vi "GetPathFromTimeStamp.vi"(2 "UTC Time":bool=TRUE, 7 "LocalTimeStamp":dbl, 13 "Changement de date à midi ?":bool=TRUE) -> (6 "Date String":string, 10 "Time String":string)   [LabVIEW 2011]
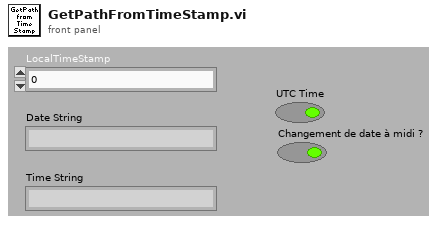
[diagram p1: front panel]
types:
  T1 = typedef "LVDateTimeRec.ctl" = cluster{"fractional second":dbl, "second":i32, "minute":i32, "hour":i32, "day of month":i32, "month":i32, "year":i32, "day of week":i32, "day of year":i32, "DST":i32}
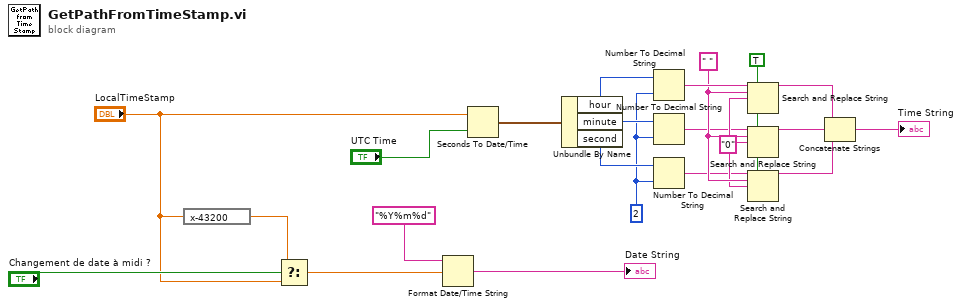
[diagram p0: block diagram]
diagram:
  w5 = 2
  w19 = TRUE ("replace all? (F)")
  w16 = "0" ("replace string (\"\")")
  w17 = " " ("search string")
  n1 = expression code="x-43200"("LocalTimeStamp") -> (w3:dbl)
  n2 = Select(t=w3, s="Changement de date à midi ?", f="LocalTimeStamp") -> (s? t:f=w1:dbl)
  n3 = Format Date/Time String(time format string (%c)="%Y%m%d", seconds (now)=w1) -> (date/time string=→"Date String":string)  [unwired: 1 in]
  n4 = Seconds To Date/Time(time stamp (now)="LocalTimeStamp", to UTC (F)="UTC Time") -> (date time rec=w12:T1)
  n5 = Unbundle By Name(w12) -> ("hour"=w10:i32, "minute"=w11:i32, "second"=w9:i32)
  n6 = Number To Decimal String(number=w10, width (-)=w5) -> (decimal integer string=w18:string)
  n7 = Number To Decimal String(number=w11, width (-)=w5) -> (decimal integer string=w15:string)
  n8 = Number To Decimal String(number=w9, width (-)=w5) -> (decimal integer string=w14:string)
  n9 = Search and Replace String(replace all?=w19, input string=w18, search string=w17, replace string=w16) -> (result string=w7:string)  [unwired: 4 in, 3 out]
  n10 = Search and Replace String(replace all?=w19, input string=w15, search string=w17, replace string=w16) -> (result string=w8:string)  [unwired: 4 in, 3 out]
  n11 = Search and Replace String(replace all?=w19, input string=w14, search string=w17, replace string=w16) -> (result string=w13:string)  [unwired: 4 in, 3 out]
  n12 = Concatenate Strings(w7, w8, w13) -> (→"Time String":string)
